vi "Is Supported Input.vi"(2 "Project in":refnum<class "Project.lvclass">, 3 "Ctl Refnum":refnum<vi>) -> (0 "Supported":bool)   [LabVIEW 2015, in "CallVIStep.lvclass"]
uses:
  CallVIStep.lvclass
  Project.lvclass
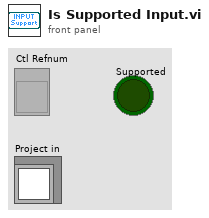
[diagram p1: front panel]
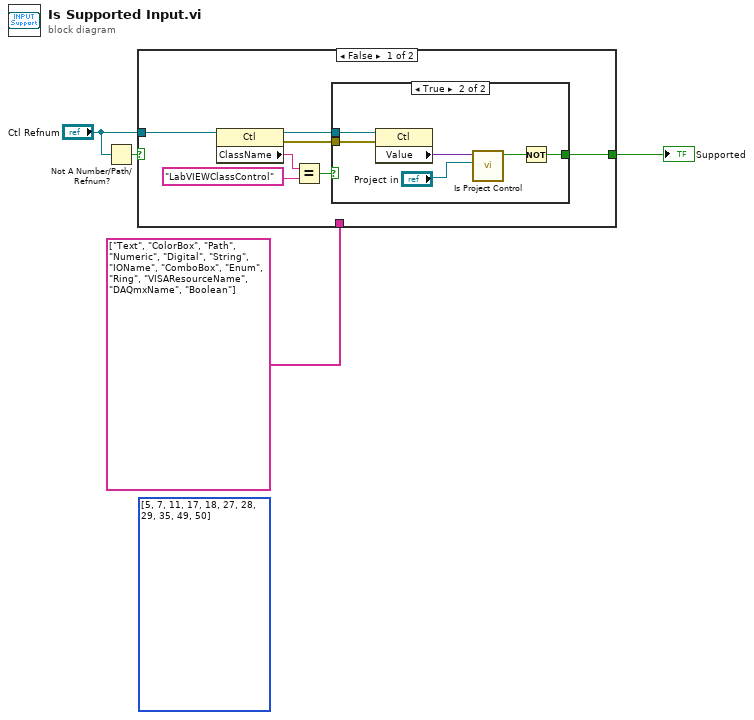
[diagram p0: block diagram]
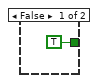
[diagram p2: hidden frame]
diagram:
  (unwired) u16[] [5, 7, 11, 17, 18, 27, 28, 29, 35, 49, 50] items=["Text"=5, "ColorBox"=7, "Path"=11, "Numeric"=17, "Digital"=18, "String"=27, "IOName"=28, "ComboBox"=29, "Enum"=35, "DAQName"=49, "VISAName"=50]
  n1 = Not A Number/Path/Refnum?(number/path/refnum="Ctl Refnum") -> (NaN/Path/Refnum?=w3:bool)
  n2 = case shown="False" w3 {
    tunnel: string[] ["Text", "ColorBox", "Path", "Numeric", "Digital", "String", "IOName", "ComboBox", "Enum", "Ring", "VISAResourceName", "DAQmxName", "Boolean"] ("Strings []") -> [_ _]
    tunnel: "Ctl Refnum" -> [w11 _]
    tunnel: [w5 _] -> w2
    frame False {
      n3 = property class="Ctl"(reference=w11) -> (reference out=w7:refnum<vi>, error out=w6:errorcluster, "ClassName"=w9:string)  [unwired: 1 in]
      n4 = Equal?(x=w9, y="LabVIEWClassControl") -> (x = y?=w8:bool)
      n5 = case shown="True" w8 {
        tunnel: w7 -> [_ w18]
        tunnel: w6 -> [_ w17]
        tunnel: [TRUE w14] -> w5
        frame False {
        }
        frame True {
          n6 = property class="Ctl"(reference=w18, error in=w17) -> ("Value"=w16:variant)  [unwired: 2 out]
          n7 = call "Is Project Control.vi"("Project"="Project in", "Control Value"=w16) -> ("Is Project Control"=w15:bool)  [unwired: 8 in, 1 out]
          n8 = Not(x=w15) -> (.not. x?=w14:bool)
        }
      }
    }
    frame True {
    }
  }
  "Supported" <- w2
